vi "img Reader Example.vi"() -> ()   [LabVIEW 2024]
uses:
  <vilib>/RTI DDS Toolkit/Types/RTI DDS Advanced Reader Configuration.ctl
  <vilib>/RTI DDS Toolkit/Types/RTI DDS ContentFilteredTopic Info.ctl
  <vilib>/RTI DDS Toolkit/Types/DDS Duration.ctl
  <vilib>/RTI DDS Toolkit/Types/RTI DDS Read Mode.ctl
  <vilib>/RTI DDS Toolkit/Types/DDS Sample Info.ctl
  <vilib>/RTI DDS Toolkit/Library/LVDDS_library.lvlib
panel:
  out "DDS Sample Info":T1
  out "Read Sample":cluster{"img":u8[], "frame_rate":dbl}
  in  "LVDDS_Read_Mode":T2
  in  "Only New Samples":bool
  out "Timeout":bool
  in  "Blocking Timeout":T3
  in  "Sample Type":cluster{"img":u8[], "frame_rate":dbl}
  in  "ContentFilteredTopic Info":T4={"Filter Type"="DDS_SQLFILTER_NAME", "ContentFilteredTopic Name"="", "Filter Expression"=""}
  in  "Advanced Reader Configuration":T5
  in  "error in (no error)":errorcluster
  in  "Stop Reading":bool
  # "Source Timestamp"
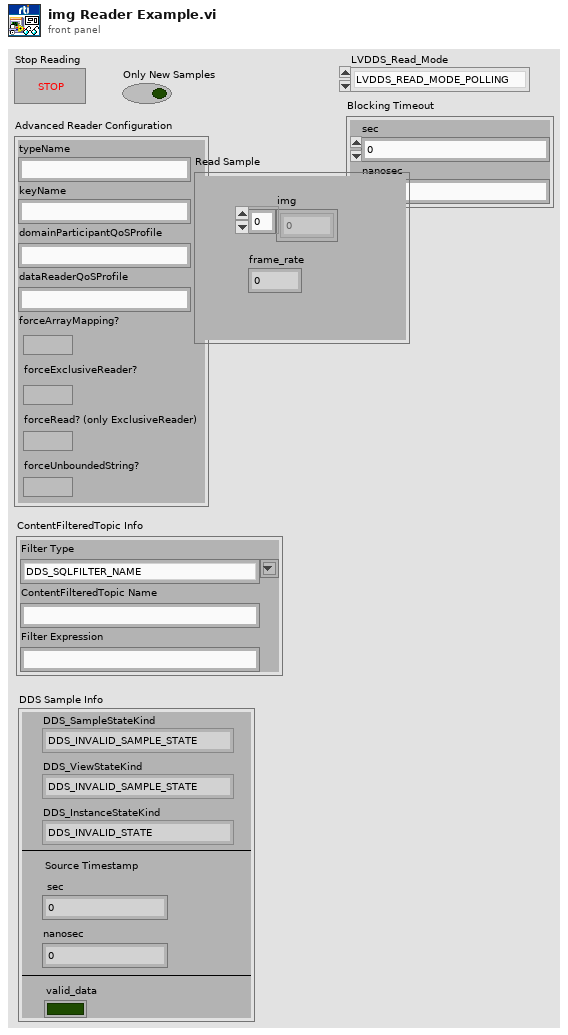
[diagram p1: front panel]
types:
  T1 = typedef "LVDDS_library.lvlib/DDS Sample Info.ctl" = cluster{"DDS_SampleStateKind":enum32{"DDS_INVALID_SAMPLE_STATE", "DDS_READ_SAMPLE_STATE", "DDS_NOT_READ_SAMPLE_STATE"}, "DDS_ViewStateKind":enum32{"DDS_INVALID_SAMPLE_STATE", "DDS_NEW_VIEW_STATE", "DDS_NOT_NEW_VIEW_STATE"}, "DDS_InstanceStateKind":enum32{"DDS_INVALID_STATE", "DDS_ALIVE_INSTANCE_STATE", "DDS_NOT_ALIVE_DISPOSED_INSTANCE_STATE", "", "DDS_NOT_ALIVE_NO_WRITERS_INSTANCE_STATE"}, "sec":i32, "nanosec":u32, "valid_data":bool}
  T2 = typedef "LVDDS_library.lvlib/RTI DDS Read Mode.ctl" = enum32{"LVDDS_READ_MODE_POLLING", "LVDDS_READ_MODE_BLOCKING"}
  T3 = typedef "LVDDS_library.lvlib/DDS Duration.ctl" = cluster{"sec":i32, "nanosec":u32}
  T4 = typedef "LVDDS_library.lvlib/RTI DDS ContentFilteredTopic Info.ctl" = cluster{"Filter Type":string, "ContentFilteredTopic Name":string, "Filter Expression":string}
  T5 = typedef "LVDDS_library.lvlib/RTI DDS Advanced Reader Configuration.ctl" = cluster{"typeName":string, "keyName":string, "domainParticipantQoSProfile":string, "dataReaderQoSProfile":string, "forceArrayMapping?":bool, "forceExclusiveReader?":bool, "forceRead? (only ExclusiveReader)":bool, "forceUnboundedString?":bool}
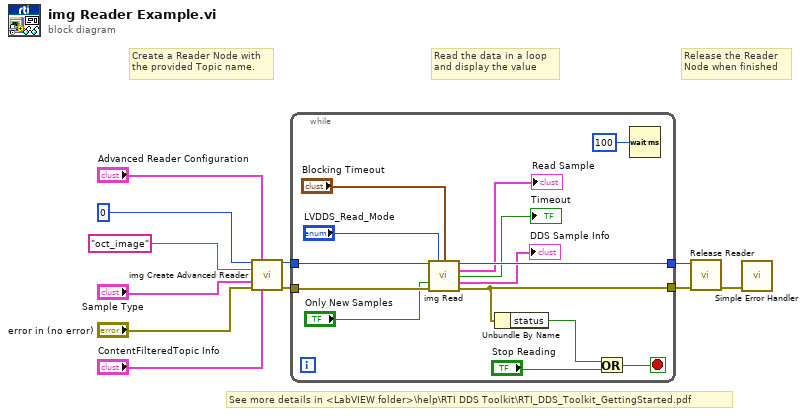
[diagram p0: block diagram]
diagram:
  # "See more details in <LabVIEW folder>\\help\\RTI DDS Toolkit\\RTI_DDS_Toolkit_GettingStarted.pdf"
  # "Release the Reader \nNode when finished"
  # "Read the data in a loop \nand display the value"
  # "Create a Reader Node with\nthe provided Topic name."
  n1 = call "img Create Advanced Reader.vi"("Domain Id"=u32 0, "Advanced Reader Configuration"="Advanced Reader Configuration", "Topic Name"="oct_image", "MyComplexType type"="Sample Type", "error in (no error)"="error in (no error)", "ContentFilteredTopic Info"="ContentFilteredTopic Info") -> ("DDS Object Ref"=w8:u64, "error out"=w7:errorcluster)  [unwired: 8 in]
  n2 = while "Main Loop" {
    tunnel: w8 -> [w25]
    tunnel: [w23] -> w11
    tunnel: w7 -> [w22]
    tunnel: [w18] -> w10
    stop <- w19 stop-if-true
    n3 = call "img Read.vi"("DDS Object Ref in"=w25, "Read Mode"="LVDDS_Read_Mode", "Blocking Timeout"="Blocking Timeout", "Only New Samples"="Only New Samples", "error in (no error)"=w22) -> ("DDS Object Ref out"=w23:u64, "Read Sample"=→"Read Sample":cluster{"img":u8[], "frame_rate":dbl}, "Timeout"=→"Timeout":bool, "DDS Sample Info"=→"DDS Sample Info":T1, "error out"=w18:errorcluster)  [unwired: 6 in]
    n4 = Unbundle By Name(w18) -> ("status"=w21:bool)
    n5 = Or(x=w21, y="Stop Reading") -> (x .or. y?=w19:bool)
    n6 = Wait (ms)(milliseconds to wait=u32 100 ("millisecond multiple")) -> ()  [unwired: 1 out]
  }
  n7 = call <vilib>:"Release Reader.vi"("error in (no error)"=w10, "DDS Object Ref"=w11) -> ("error out"=w9:errorcluster)  [unwired: 9 in]
  n8 = call <vilib>:"Simple Error Handler.vi"("error in (no error)"=w9) -> ()  [unwired: 4 in, 5 out]
